vi "Config Voltage Range.vi"(0 "VISA resource name":refnum<visa-resource-name>, 5 "V Range (6: 600V)":u16(ring)=6 items=["Auto", "15V", "30V", "60V", "150V", "300V", "600V"], 11 "error in (no error)":errorcluster) -> (4 "VISA resource name out":refnum<visa-resource-name>, 15 "error out":errorcluster)   [LabVIEW 2019, in "Yokogawa WT200 Series.lvlib"]
doc: "This VI sends the voltage range commands to the WT200 Series."
uses:
  Yokogawa WT200 Series.lvlib
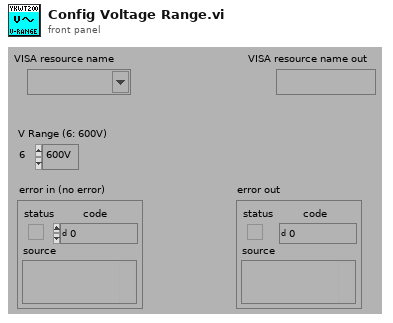
[diagram p1: front panel]
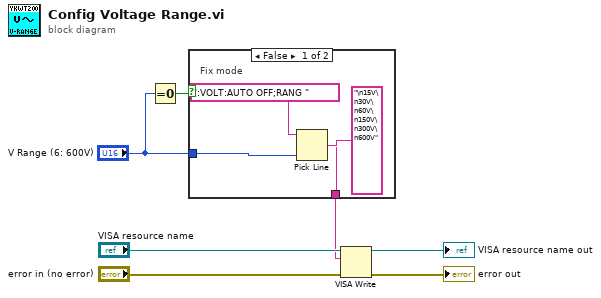
[diagram p0: block diagram]
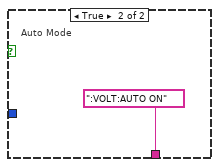
[diagram p2: hidden frame]
diagram:
  n1 = Equal To 0?(x="V Range (6: 600V)") -> (x = 0?=w7:bool)
  n2 = case shown="False" w7 {
    tunnel: [w10 ":VOLT:AUTO ON"] -> w1
    tunnel: "V Range (6: 600V)" -> [w8 _]
    frame False {
      # "Fix mode"
      n3 = Pick Line(string ("")=":VOLT:AUTO OFF;RANG ", multi-line string="\n15V\n30V\n60V\n150V\n300V\n600V", line index=w8) -> (output string=w10:string)
    }
    frame True {
      # "Auto Mode"
    }
  }
  n4 = VISA Write(VISA resource name="VISA resource name", write buffer=w1, error in (no error)="error in (no error)") -> (VISA resource name out=→"VISA resource name out":refnum<visa-resource-name>, error out=→"error out":errorcluster)  [unwired: 1 out]
